vi "Write Header and Footer [ ].vi"(8 "error in (no error)":errorcluster, 10 "Header and Footer [ ]":T1, 11 "Header and Footer Class in":refnum<class "Header and Footer Class.lvclass">) -> (0 "error out":errorcluster, 3 "Header and Footer Class out":refnum<class "Header and Footer Class.lvclass">)   [LabVIEW 2019, in "Header and Footer Class.lvclass"]
uses:
  <userlib>/Exaprom PDF/LV Class/Header and Footer Class/Header and Footer Class.lvclass
  <userlib>/Exaprom PDF/LV Class/Header and Footer Class/VIs/Controls/Header Footer [ ] V2.ctl
  <userlib>/Exaprom PDF/LV Class/Header and Footer Class/VIs/Controls/Header Footer cluster V2.ctl
  <userlib>/Exaprom PDF/Controls/Header, Footer and Watermark Controls/Header or Footer.ctl
  <userlib>/Exaprom PDF/Controls/Header, Footer and Watermark Controls/Header Footer Type.ctl
  <userlib>/Exaprom PDF/Controls/Header, Footer and Watermark Controls/Header footer horiz alignment.ctl
  <userlib>/Exaprom PDF/Controls/Table Controls/Cell Vertical alignment.ctl
  <userlib>/Exaprom PDF/Controls/Text Controls/Line spacing.ctl
  <userlib>/Exaprom PDF/Controls/Header, Footer and Watermark Controls/Page number.ctl
  <userlib>/Exaprom PDF/Controls/Font Controls/Font complete cluster horizontal.ctl
  <userlib>/Exaprom PDF/Controls/Font Controls/Font size.ctl
  <userlib>/Exaprom PDF/Controls/Font Controls/Font color.ctl
  <userlib>/Exaprom PDF/Controls/Font Controls/Type and encoding.ctl
  <userlib>/Exaprom PDF/Controls/Text Controls/Unicode/Type and run direction.ctl
  C:/Program Files/National Instruments/LabVIEW 2019/user.lib/Exaprom PDF/DLL/itextsharp.dll
  DLL/itextsharp.dll
  <userlib>/Exaprom PDF/Controls/Header, Footer and Watermark Controls/Header Footer Line.ctl
  <userlib>/Exaprom PDF/LV Class/Header and Footer Class/Header and Footer Class.lvclass/Header and Footer Class.ctl
panel:
  # "X"
  # "Y"
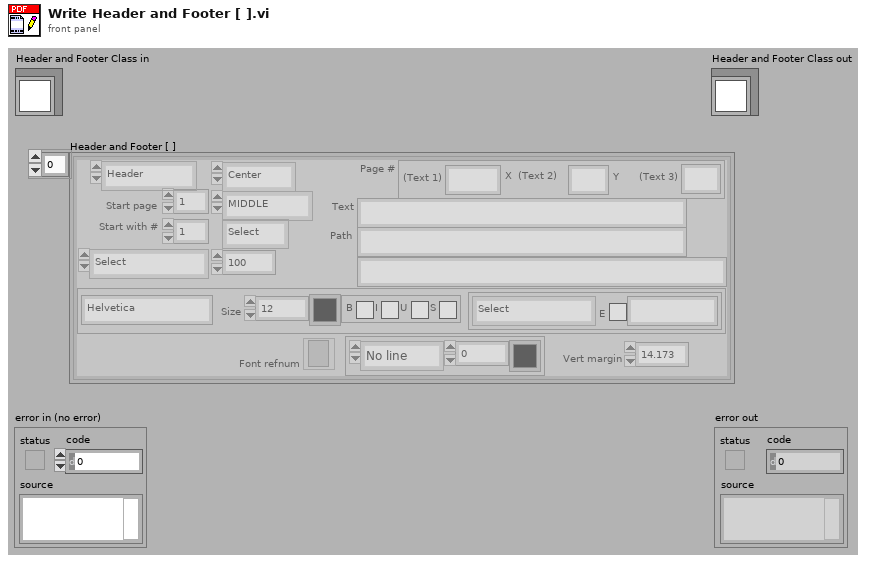
[diagram p1: front panel]
types:
  T1 = typedef "Header Footer [ ] V2.ctl" = T2[]
  T2 = typedef "Header Footer cluster V2.ctl" = cluster{"Header or Footer":T3, "Start page":i32, "Start with #":i32, "Type":T4, "Alignment":T5, "Vertical Alignement":T6, "Line spacing":T7, "Image (%)":sgl, "Page #":T8, "Text":string, "Path":string, "Font":T9, "Font refnum":refnum<k24>, "Line":cluster{"Line":T14, "Thickness (points)":sgl, "Colour":T11}, "Vert margin":dbl, "Hyperlink":string}
  T3 = typedef "Header or Footer.ctl" = enum16{"Header", "Footer"}
  T4 = typedef "Header Footer Type.ctl" = enum16{"Select", "Text", "Text + hyperlink", "Page number", "Image", "Image + hyperlink"}
  T5 = typedef "Header footer horiz alignment.ctl" = enum16{"Left", "Center", "Right"}
  T6 = typedef "Cell Vertical alignment.ctl" = enum16{"TOP", "MIDDLE", "BOTTOM"}
  T7 = typedef "Line spacing.ctl" = enum16{"Select", "1.0", "1.5", "2.0"}
  T8 = typedef "Page number.ctl" = cluster{"Text 1":string, "Text 2":string, "Text 3":string}
  T9 = typedef "Font complete cluster horizontal.ctl" = cluster{"Name":string, "Size":T10, "Color":T11, "Style":cluster{"Bold":bool, "Italic":bool, "Underline":bool, "Strikeout":bool}, "Type":T12}
  T10 = typedef "Font size.ctl" = sgl
  T11 = typedef "Font color.ctl" = u32
  T12 = typedef "Type and encoding.ctl" = cluster{"Type&direction":T13, "Embedded":bool, "Encoding":string}
  T13 = typedef "Type and run direction.ctl" = enum16{"Select", "ASCII", "UTF-16", "UTF-16 (default)", "UTF-16 (LTR)", "UTF-16 (RTL)"}
  T14 = typedef "Header Footer Line.ctl" = enum16{"No line", "Horizontal line"}
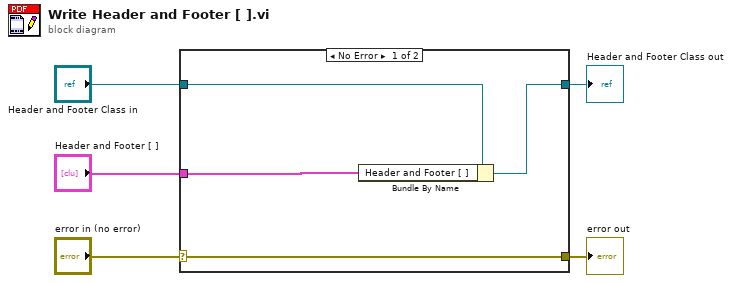
[diagram p0: block diagram]
diagram:
  n1 = case shown="No Error" "error in (no error)" {
    selector: "error in (no error)" -> [w9 w10]
    tunnel: [w9 w10] -> w4
    tunnel: [w7 w11] -> w2
    tunnel: "Header and Footer Class in" -> [w8 w11]
    tunnel: "Header and Footer [ ]" -> [w6 _]
    frame No Error {
      n2 = Bundle By Name(cluster=w8, "Header and Footer [ ]"=w6) -> (w7:refnum<class "Header and Footer Class.lvclass">)
    }
    frame Error {
    }
  }
  "error out" <- w4
  "Header and Footer Class out" <- w2
